vi "Scripting_GetClassPathFromControlRef.vi"(10 "ViRef":refnum<vi>, 11 "Control in":refnum<vi>) -> (3 "class path":path)   [LabVIEW 2020, in "Scripting.lvclass"]
uses:
  <resource>/Framework/Providers/Open_GDS/ClassProviders/Common/ScriptingFunctions/Scripting.lvclass
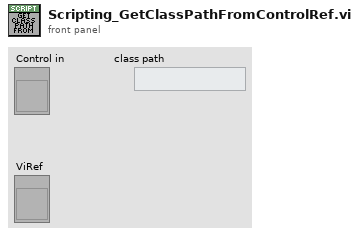
[diagram p1: front panel]
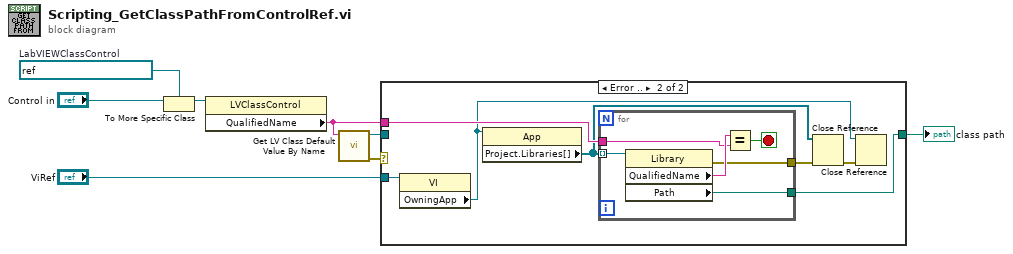
[diagram p0: block diagram]
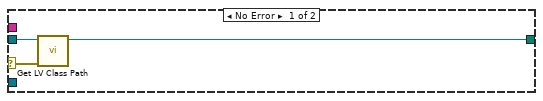
[diagram p2: hidden frame]
diagram:
  w5 = refnum<vi> refnum  # LabVIEWClassControl
  n1 = To More Specific Class(target class=w5, reference="Control in") -> (specific class reference=w8:refnum<vi>)  [unwired: 1 in, 1 out]
  n2 = property class="LVClassControl"(reference=w8) -> ("QualifiedName"=w1:string)  [unwired: 1 in, 2 out]
  n3 = call <vilib>:"Get LV Class Default Value By Name.vi"("class name"=w1) -> ("error out"=w7:errorcluster, "object"=w6:refnum<class>)  [unwired: 9 in]
  n4 = case shown="Error .." w7 {
    selector: w7 -> [w11 _]
    tunnel: w6 -> [w10 _]
    tunnel: [w9 w16] -> w3
    tunnel: "ViRef" -> [_ w18]
    tunnel: w1 -> [_ w17]
    frame No Error {
      n5 = call <vilib>:"Get LV Class Path.vi"("error in (no error)"=w11, "object"=w10) -> ("class path"=w9:path)  [unwired: 8 in, 1 out]
    }
    frame Error {
      n6 = property class="VI"(reference=w18) -> ("OwningApp"=w12:refnum<vi>)  [unwired: 1 in, 2 out]
      n7 = property class="App"(reference=w12) -> ("Project.Libraries[]"=w15:refnum<vi>[])  [unwired: 1 in, 2 out]
      n8 = for {
        tunnel: w15 -> [w24] mode=indexing
        tunnel: w17 -> [w22]
        tunnel: [w20] -> w16
        tunnel: [w19] -> w14
        stop <- w21 stop-if-true
        n9 = property class="Library"(reference=w24) -> (error out=w19:errorcluster, "QualifiedName"=w23:string, "Path"=w20:path)  [unwired: 1 in, 1 out]
        n10 = Equal?(x=w23, y=w22) -> (x = y?=w21:bool)
      }
      n11 = Close Reference(reference=w15, error in (no error)=w14) -> (error out=w13:errorcluster)
      n12 = Close Reference(reference=w12, error in (no error)=w13) -> ()  [unwired: 1 out]
    }
  }
  "class path" <- w3
